vi "Compare Received Data with File.vi"() -> ()   [LabVIEW 2019]
doc: "This example program configures the first available ARINC 429\nReceive and Transmit Channels on the specified card. The TX\nChannel is scheduled with a single Label message. The RX Channel is\nconfigured to this same Label using a List Buffer. The TX List Buffer\nis loaded with data from a file. The data field from the received word is\ncompared with the data from the same file. The number of Messages\nwith matching data is displayed along with the number of Messages\nwith data errors. The XML configuration enables the internal Self Test\nBus, so no external connections are required."
uses:
  <instrlib>/BTICardLib/Private/Initialize By Card Number and Core Number.vi
  <instrlib>/BTI429Lib/Private/Rx/Configure/Configure Rx Channel From XML.vi
  <instrlib>/BTI429Lib/Private/Rx/Configure/Get Rx Label Handle Name.vi
  <instrlib>/BTI429Lib/Private/Tx/Configure/Configure Tx Channel From XML.vi
  <instrlib>/BTI429Lib/Private/Utility/Set Fld Value.vi
  <instrlib>/BTI429Lib/Private/Tx/Data/Set Scheduled Message List Data Dynamic.vi
  <instrlib>/BTI429Lib/Private/Core/Action-Status/Start All Channels.vi
  <instrlib>/BTI429Lib/Private/Utility/Get Fld Value.vi
  <instrlib>/BTI429Lib/Private/Core/Action-Status/Stop All Channels.vi
  <instrlib>/BTICardLib/BTICardLV.lvlib
  <instrlib>/BTI429Lib/BTI429LV.lvlib
panel:
  out "Total Size":i32
  out "Current Position":u32
  out "TX channel number":i32
  in  "TX Channel Config":string="TX Channel Config.XML"
  out "Data Errors":i32
  out "Matches":i32
  out "core number":i32
  in  "Data Filename":string="Data File.txt"
  out "RX channel number":i32
  in  "RX Channel Config":string="RX Channel Config.XML"
  in  "stop":bool
  out "error out":errorcluster
  in  "Card Number":i32
  # "ARINC 429: Compare Received Data with File"
  # "©2016 Astronics Ballard Technology"
  # "This example program configures the first available ARINC 429\nReceive and Transmit Channels on the specified card. The TX\nChannel is scheduled with a single Label message. The RX Channel is\nconfigured  to this same Label using a List Buffer. The TX List Buffer\nis loaded with data from a file. The data field from the received word is\ncompared with the data from the same file. The number of Messages\nwith matching data is displayed along with the number of Messages\nwith data errors. The XML configuration enables the internal Self Test\nBus, so no external connections are required."
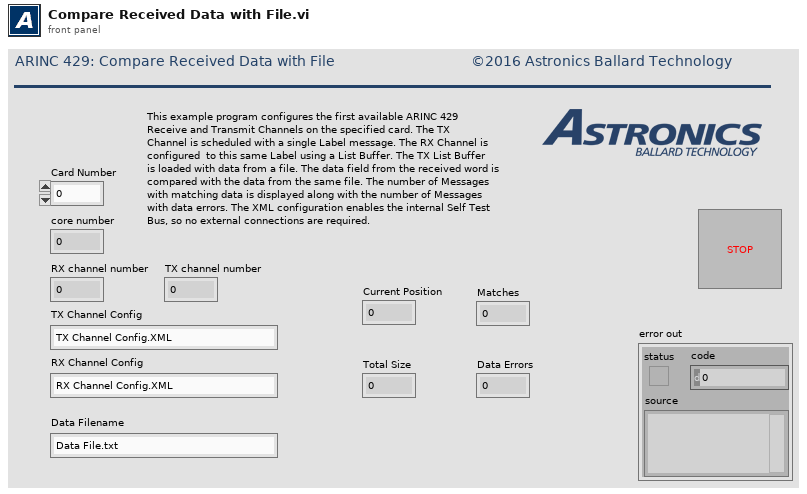
[diagram p1: front panel]
types:
  T1 = enum16{"open", "replace", "create", "open or create", "replace or create", "replace or create with confirmation"}
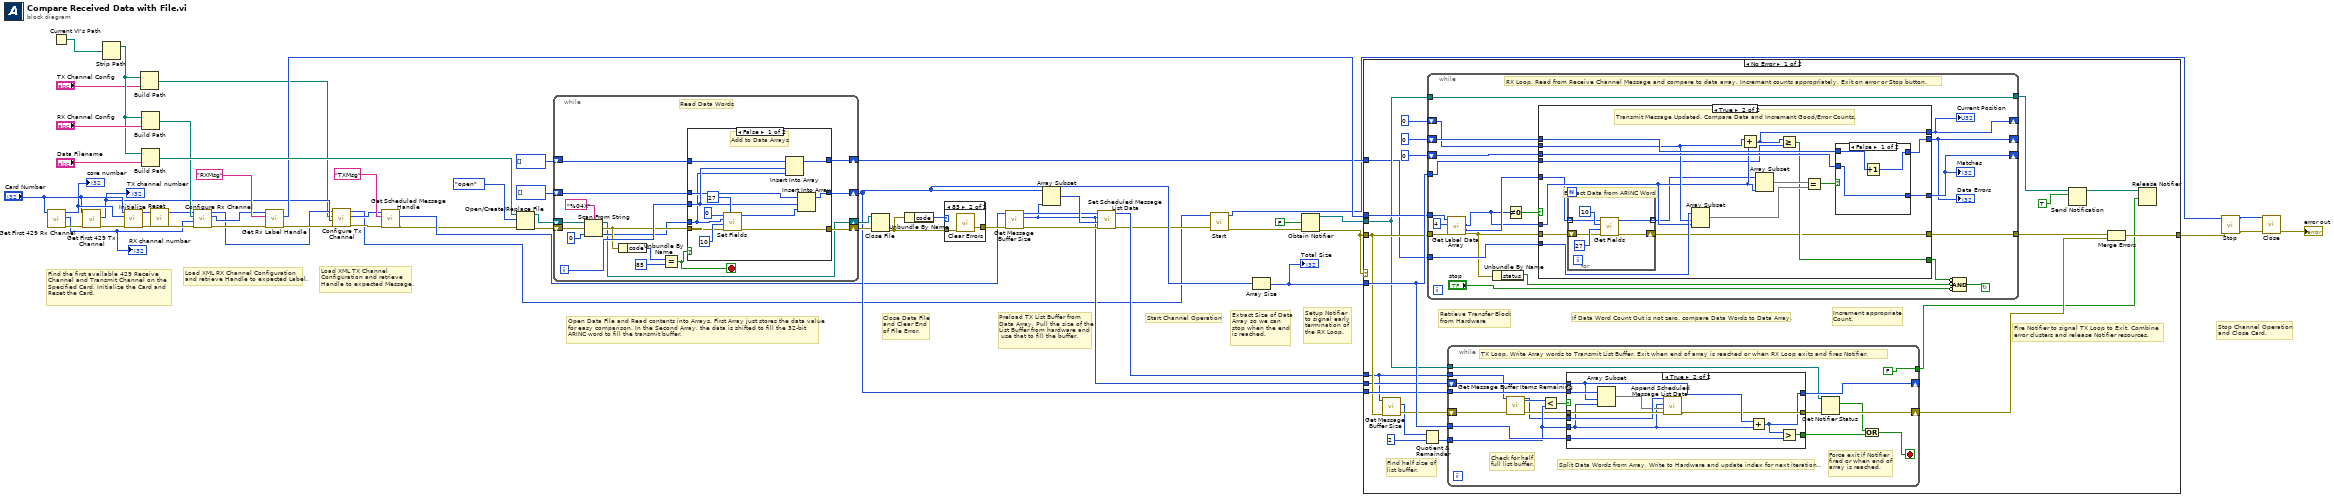
[diagram p0: block diagram]
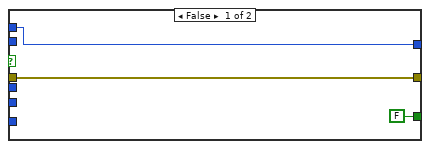
[diagram p3: hidden frame]
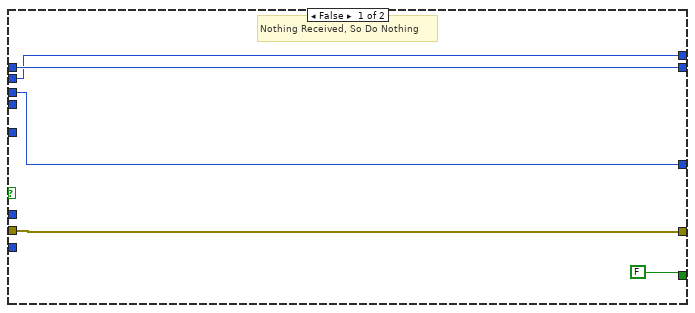
[diagram p4: hidden frame]
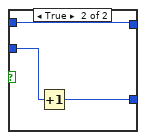
[diagram p5: hidden frame]
diagram:
  # "Load XML TX Channel\nConfiguration and retrieve\nHandle to expected Message."
  # "Setup Notifier\nto signal early\ntermination of \nthe RX Loop."
  # "Extract Size of Data\nArray so we can\nstop when the end\nis reached."
  # "Start Channel Operation"
  # "Preload TX List Buffer from\nData Array. Pull the size of the\nList Buffer from hardware and\n use that to fill the buffer."
  # "Close Data File\nand Clear End\nof File Error."
  # "Open Data File and Read contents into Arrays. First Array just stores the data value\nfor easy comparison. In the Second Array, the data is shifted to fill the 32-bit\nARINC word to fill the transmit buffer."
  # "Stop Channel Operation\nand Close Card."
  # "Load XML RX Channel Configuration\nand retrieve Handle to expected Label."
  # "Find the first available 429 Receive Channel and Transmit Channel on the Specified Card, Initialize the Card and\nReset the Card."
  n1 = call "Get First 429 Rx Channel.vi"("Card Number"="Card Number") -> ("error out"=w42:errorcluster, "Channel Number"=w35:i32, "Core Number"=w41:i32)  [unwired: 8 in]
  "RX channel number" <- w35
  "core number" <- w41
  n2 = Current VI's Path() -> (path=w54:path)
  n3 = call "Get First 429 Tx Channel.vi"("error in (no error)"=w42, "Card Number"="Card Number") -> ("error out"=w43:errorcluster, "Channel Number"=w30:i32)  [unwired: 7 in, 1 out]
  "TX channel number" <- w30
  n4 = Strip Path(path=w54) -> (stripped path=w17:path)  [unwired: 1 out]
  n5 = call-poly <instrlib>:"Initialize.vi"("error in (no error)"=w43, "core number"=w41, "card number"="Card Number") -> ("error out"=w58:errorcluster, "core handle out"=w57:u64)  [unwired: 7 in]
  n6 = Build Path(base path=w17, name or relative path="TX Channel Config") -> (appended path=w18:path)
  n7 = Build Path(base path=w17, name or relative path="RX Channel Config") -> (appended path=w34:path)
  n8 = Build Path(base path=w17, name or relative path="Data Filename") -> (appended path=w51:path)
  n9 = call <instrlib>:"Reset.vi"("error in (no error)"=w58, "core handle in"=w57) -> ("error out"=w36:errorcluster, "core handle out"=w33:u64)  [unwired: 8 in]
  n10 = call-poly <instrlib>:"Configure Rx Channel.vi"("error in (no error)"=w36, "channel number in"=w35, "configuration file path"=w34, "core handle in"=w33) -> ("error out"=w37:errorcluster, "channel handle out"=w32:u64, "core handle out"=w29:u64)  [unwired: 5 in]
  n11 = call-poly <instrlib>:"Get Rx Label Handle.vi"("error in (no error)"=w37, "label name"="RXMsg", "channel handle in"=w32) -> ("error out"=w31:errorcluster, "label handle out"=w38:u64)  [unwired: 6 in, 1 out]
  n12 = call-poly <instrlib>:"Configure Tx Channel.vi"("error in (no error)"=w31, "channel number in"=w30, "configuration file path"=w18, "core handle in"=w29) -> ("error out"=w28:errorcluster, "channel handle out"=w26:u64, "core handle out"=w4:u64)  [unwired: 5 in]
  n13 = call <instrlib>:"Get Scheduled Message Handle.vi"("error in (no error)"=w28, "message name"="TXMsg" ("rt transfer name"), "channel handle in"=w26) -> ("error out"=w6:errorcluster, "message handle out"=w7:u64)  [unwired: 6 in, 1 out]
  n14 = Open/Create/Replace File(file path (use dialog)=w51, error in=w6, operation (0:open)=T1."open") -> (refnum out=w49:refnum<file>, error out=w50:errorcluster)  [unwired: 3 in, 1 out]
  n15 = while {
    shift-right: [w61] -> w47
    shift-left: w49 -> [w72]
    shift-right: [w63] -> w48
    shift-left: w50 -> [w71]
    shift-right: [w66] -> w9
    shift-left: u32[] [] -> [w67]
    shift-right: [w60] -> w8
    shift-left: u32[] [] -> [w59]
    i -> [w65]
    stop <- w68 stop-if-true
    # "Read Data Words"
    n16 = Scan From String("%04X" ("format string"), w72, w71, default 1=u32 0 ("default value 1")) -> (w61:refnum<file>, w64:errorcluster, output 1=w62:u32)
    n17 = Unbundle By Name(w64) -> ("code"=w69:i32)
    n18 = Equal?(x=w69, y=85) -> (x = y?=w68:bool)
    n19 = case shown="False" w68 {
      tunnel: w67 -> [w78 w89]
      tunnel: [w86 w89] -> w66
      tunnel: w65 -> [w79 _]
      tunnel: w64 -> [w82 w88]
      tunnel: [w76 w88] -> w63
      tunnel: w62 -> [w77 _]
      tunnel: [w81 w87] -> w60
      tunnel: w59 -> [w80 w87]
      frame False {
        # "Add to Data Arrays"
        n20 = call-poly <instrlib>:"Set Fields.vi"("end bit"=u16 27, "error in (no error)"=w82, "start bit"=u16 10, "data"=w77, "message"=u32 0) -> ("error out"=w76:errorcluster, "message out"=w75:u32)  [unwired: 5 in]
        n21 = Insert Into Array(array=w80, index=w79, new element=w77) -> (w81:u32[])
        n22 = Insert Into Array(array=w78, index=w79, new element=w75) -> (w86:u32[])
      }
      frame True {
        # "EOF, Do Nothing"
      }
    }
  }
  n23 = Close File(refnum=w47, error in=w48) -> (error out=w1:errorcluster)  [unwired: 1 out]
  n24 = Unbundle By Name(w1) -> ("code"=w2:i32)
  n25 = case shown="85" w2 {
    tunnel: w1 -> [w90 w92]
    tunnel: [w90 w91] -> w22
    frame 0, Default {
    }
    frame 85 {
      n26 = call <vilib>:"Clear Errors.vi"("error in (no error)"=w92) -> ("error out"=w91:errorcluster)  [unwired: 5 in, 1 out]
    }
  }
  n27 = call <instrlib>:"Get Message Buffer Size.vi"("error in (no error)"=w22, "message handle in"=w7) -> ("error out"=w25:errorcluster, "total size of buffer"=w11:i32, "message handle out"=w23:u64)  [unwired: 7 in]
  n28 = Array Subset(array=w9, length=w11) -> (w24:u32[])  [unwired: 1 in]
  n29 = call-poly <instrlib>:"Set Scheduled Message List Data.vi"("error in (no error)"=w25, "values"=w24, "value count"=w11, "message handle in"=w23) -> ("error out"=w5:errorcluster, "message handle out"=w19:u64)  [unwired: 6 in]
  n30 = call-poly <instrlib>:"Start.vi"("error in (no error)"=w5, "core handle in"=w4) -> ("error out"=w12:errorcluster, "core handle out"=w3:u64)  [unwired: 8 in]
  n31 = Array Size(array=w9) -> (size(s)=w45:i32)
  "Total Size" <- w45
  n32 = Obtain Notifier(notification data type=FALSE, error in (no error)=w12) -> (notifier out=w15:refnum<notifier>, error out=w13:errorcluster)  [unwired: 2 in, 1 out]
  n33 = case shown="No Error" w13 {
    tunnel: w45 -> [w109 _]
    tunnel: w38 -> [w108 _]
    tunnel: w9 -> [w107 _]
    tunnel: w13 -> [w105 w201]
    tunnel: w19 -> [w94 _]
    tunnel: w11 -> [w101 _]
    tunnel: w15 -> [w98 _]
    tunnel: [w96 w201] -> w14
    tunnel: w8 -> [w93 _]
    frame No Error {
      # "Find half size of\nlist buffer."
      # "Fire Notifier to signal TX Loop to Exit. Combine\nerror clusters and release Notifier resources."
      # "Increment appropriate\nCount."
      # "If Data Word Count Out is not zero, compare Data Words to Data Array."
      # "Retrieve Transfer Block\nfrom Hardware"
      n34 = call <instrlib>:"Get Message Buffer Size.vi"("error in (no error)"=w105, "message handle in"=w94) -> ("error out"=w106:errorcluster, "total size of buffer"=w103:i32)  [unwired: 7 in, 1 out]
      n35 = Quotient & Remainder(x=w103, y=2) -> (floor(x/y)=w102:i32)  [unwired: 1 out]
      n36 = while {
        tunnel: [w166] -> w99
        tunnel: w105 -> [w152]
        tunnel: w108 -> [w148]
        shift-right: [w162] -> _
        shift-left: 0 -> [w163]
        shift-right: [w160] -> _
        shift-left: 0 -> [w161]
        tunnel: w93 -> [w159]
        shift-right: [w157] -> _
        shift-left: 0 -> [w158]
        tunnel: w109 -> [w153]
        tunnel: w98 -> [w146]
        tunnel: [w146] -> w97
        stop <- w155 continue-if-true
        # "RX Loop. Read from Receive Channel Message and compare to data array. Increment counts appropriately. Exit on error or Stop button."
        n37 = call <instrlib>:"Get Label Data Array.vi"("error in (no error)"=w152, "data items to read"=4 ("data word count in"), "label handle in"=w148) -> ("error out"=w151:errorcluster, "data values"=w150:u32[], "data items read"=w149:u32)  [unwired: 5 in, 1 out]
        n38 = Unbundle By Name(w151) -> ("status"=w164:bool)
        n39 = Not Equal To 0?(x=w149) -> (x != 0?=w156:bool)
        n40 = case shown="True" w156 {
          tunnel: w151 -> [w171 w175]
          tunnel: [w171 w174] -> w166
          tunnel: w163 -> [w169 w188]
          tunnel: [w169 w187] -> w162
          tunnel: w161 -> [w170 w186]
          tunnel: [w170 w185] -> w160
          tunnel: w159 -> [_ w181]
          tunnel: w158 -> [w168 w180]
          tunnel: [w168 w178] -> w157
          tunnel: w149 -> [_ w179]
          tunnel: w150 -> [_ w173]
          tunnel: [FALSE w177] -> w154
          tunnel: w153 -> [_ w176]
          frame False {
            # "Nothing Received, So Do Nothing"
          }
          frame True {
            # "Transmit Message Updated. Compare Data and Increment Good/Error Counts."
            n41 = for {
              shift-right: [w191] -> w174
              shift-left: w175 -> [w192]
              tunnel: w173 -> [w190] mode=indexing
              tunnel: [w189] -> w172 mode=indexing
              # "Extract Data from ARINC Word"
              n42 = call-poly <instrlib>:"Get Fields.vi"("error in (no error)"=w192, "end bit"=u16 27 ("least significant bit"), "start bit"=u16 10 ("most significant bit"), "message"=w190) -> ("error out"=w191:errorcluster, "value out"=w189:u32)  [unwired: 6 in]
            }
            n43 = Array Subset(array=w181, index=w180, length=w179) -> (w182:u32[])
            n44 = Add(x=w180, y=w179) -> (x+y=w178:u32)
            n45 = Array Subset(array=w172, length=w179) -> (w184:u32[])  [unwired: 1 in]
            n46 = Greater Or Equal?(x=w178, y=w176) -> (x >= y?=w177:bool)
            n47 = Equal?(x=w184, y=w182) -> (x = y?=w183:bool)
            n48 = case shown="False" w183 {
              tunnel: w188 -> [w197 w200]
              tunnel: [w197 w199] -> w187
              tunnel: w186 -> [w195 w198]
              tunnel: [w196 w198] -> w185
              frame False {
                n49 = Increment(x=w195) -> (x+1=w196:i32)
              }
              frame True {
                n50 = Increment(x=w200) -> (x+1=w199:i32)
              }
            }
          }
        }
        "Matches" <- w162
        "Data Errors" <- w160
        "Current Position" <- w157
        n51 = Compound Arithmetic op=AND(invert w154, invert w164, invert "stop") -> (w155:bool)
      }
      n52 = while {
        tunnel: w107 -> [w132]
        shift-right: [w130] -> _
        shift-left: w101 -> [w131]
        tunnel: w109 -> [w129]
        shift-right: [w128] -> w111
        shift-left: w106 -> [w122]
        tunnel: w98 -> [w126]
        tunnel: w94 -> [w121]
        tunnel: w102 -> [w118]
        tunnel: [FALSE] -> w95
        stop <- w125 stop-if-true
        # "Check for half\nfull list buffer."
        # "Force exit if Notifier\nfired or when end of\narray is reached."
        # "Split Data Words from Array, Write to Hardware and update index for next iteration.."
        # "TX Loop. Write Array words to Transmit List Buffer. Exit when end of array is reached or when RX Loop exits and fires Notifier."
        n53 = call <instrlib>:"Get Message Buffer Items Remaining.vi"("error in (no error)"=w122, "message handle in"=w121) -> ("error out"=w117:errorcluster, "buffer items remaining"=w119:i32, "message handle out"=w116:u64)  [unwired: 7 in]
        n54 = Less?(x=w119, y=w118) -> (x < y?=w120:bool)
        n55 = case shown="True" w120 {
          tunnel: w132 -> [_ w145]
          tunnel: w131 -> [w135 w142]
          tunnel: [w135 w136] -> w130
          tunnel: w129 -> [_ w144]
          tunnel: [w134 w141] -> w127
          tunnel: [FALSE w143] -> w124
          tunnel: w118 -> [_ w137]
          tunnel: w117 -> [w134 w140]
          tunnel: w116 -> [_ w139]
          frame False {
          }
          frame True {
            n56 = Array Subset(array=w145, index=w142, length=w137) -> (w138:u32[])
            n57 = call <instrlib>:"Append Scheduled Message List Data.vi"("error in (no error)"=w140, "values"=w138, "value count"=w137, "message handle in"=w139) -> ("error out"=w141:errorcluster)  [unwired: 6 in, 1 out]
            n58 = Add(x=w142, y=w137) -> (x+y=w136:i32)
            n59 = Greater?(x=w136, y=w144) -> (0:w143:bool)
          }
        }
        n60 = Get Notifier Status(notifier=w126, error in (no error)=w127) -> (current notification=w123:bool, error out=w128:errorcluster)  [unwired: 3 out]
        n61 = Or(x=w123, y=w124) -> (x .or. y?=w125:bool)
      }
      n62 = Send Notification(notification=TRUE, notifier=w97) -> (notifier out=w110:refnum<notifier>)  [unwired: 1 in, 1 out]
      n63 = Merge Errors(w99, w111) -> (w96:errorcluster)
      n64 = Release Notifier(notifier=w110, force destroy? (F)=w95) -> ()  [unwired: 1 in, 3 out]
    }
    frame Error {
    }
  }
  n65 = call-poly <instrlib>:"Stop.vi"("error in (no error)"=w14, "core handle in"=w3) -> ("error out"=w21:errorcluster, "core handle out"=w20:u64)  [unwired: 8 in]
  n66 = call <instrlib>:"Close.vi"("error in (no error)"=w21, "core handle in"=w20) -> ("error out"=→"error out":errorcluster)  [unwired: 8 in, 1 out]
